vi "SetDCBias_example.vi"() -> ()   [LabVIEW 2012]
panel:
  in  "State (F: Off)":bool
  in  "stop":bool
  in  "Voltage Level (V) (0.0)":dbl
  in  "VISA resource name":refnum<visa-resource-name>
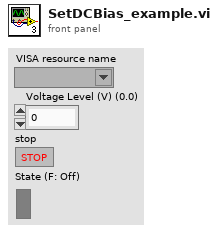
[diagram p1: front panel]
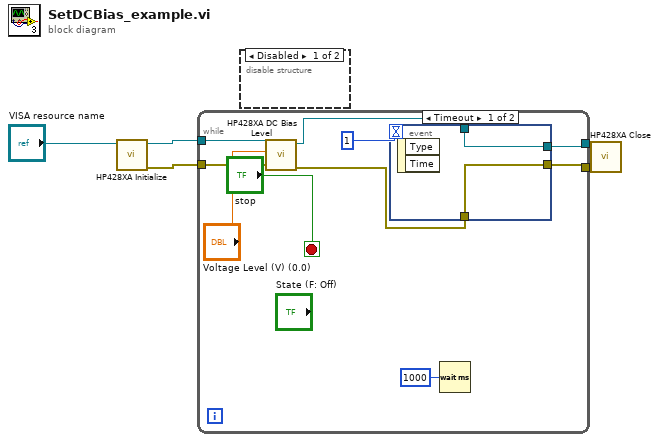
[diagram p0: block diagram]
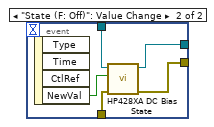
[diagram p2: hidden frame]
diagram:
  n1 = call <instrlib>:"HP428XA Initialize.vi"("VISA resource name"="VISA resource name") -> ("error out"=w4:errorcluster, "VISA session"=w5:refnum<visa-resource-name>)  [unwired: 9 in]
  n2 = while {
    tunnel: w5 -> [w15]
    tunnel: w4 -> [w14]
    tunnel: [w6] -> w3
    tunnel: [w7] -> w2
    stop <- "stop" stop-if-true
    n3 = call <instrlib>:"HP428XA DC Bias Level.vi"("error in (no error)"=w14, "Voltage Level (V) (0.0)"="Voltage Level (V) (0.0)", "VISA session"=w15) -> ("error out"=w8:errorcluster, "dup VISA session"=w9:refnum<visa-resource-name>)  [unwired: 7 in]
    n4 = event shown="[0] Timeout" {
      selector: _ -> [_ _]
      dyn-events: _ -> [_ _]
      timeout: 1 -> [_ _]
      tunnel: w9 -> [w16 w21]
      tunnel: w8 -> [w17 w20]
      tunnel: [w17 w19] -> w7
      tunnel: [w16 w18] -> w6
      event Timeout {
        n5 = event-data() -> ()  [unwired: 1 in, 2 out]
      }
      event "State (F: Off)": Value Change {
        n6 = event-data() -> ("NewVal"=w22:bool)  [unwired: 1 in, 3 out]
        n7 = call <instrlib>:"HP428XA DC Bias State.vi"("error in (no error)"=w20, "State (F: Off)"=w22, "VISA session"=w21) -> ("error out"=w19:errorcluster, "dup VISA session"=w18:refnum<visa-resource-name>)  [unwired: 7 in]
      }
    }
    n8 = Wait (ms)(milliseconds to wait=u32 1000) -> ()  [unwired: 1 out]
  }
  n9 = disable-structure shown="Disabled" {
    frame Disabled {
    }
    frame Enabled {
    }
  }
  n10 = call <instrlib>:"HP428XA Close.vi"("error in (no error)"=w2, "VISA session"=w3) -> ()  [unwired: 9 in, 1 out]
